vi "FB_MFA_SetMotorFeedback_Type1.vi"(11 "SetMotorFeedbackType":i16) -> (2 "MotorFeedback":i16, 3 "MotFbError":bool)   [LabVIEW 2011]
panel:
  out "error MotorFeedbackGet":errorcluster
  out "error MotorFeedBackPut":errorcluster
  out "AAABuild":i32
  in  "MintController":refnum<k7>(container)
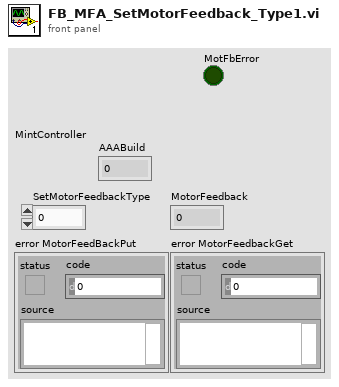
[diagram p1: front panel]
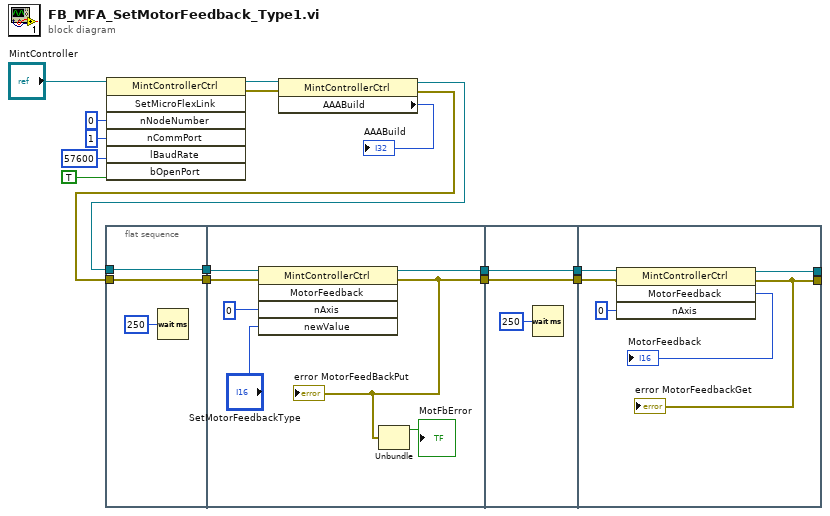
[diagram p0: block diagram]
diagram:
  n1 = flat-sequence {
    tunnel: [w19] -> w6
    tunnel: [w18] -> w5
    tunnel: w8 -> [w19]
    tunnel: w7 -> [w18]
    tunnel: w6 -> [w25]
    tunnel: w5 -> [w24]
    tunnel: [w23] -> w4
    tunnel: [w21] -> w3
    tunnel: w4 -> [w29]
    tunnel: w3 -> [w28]
    tunnel: [w29] -> w2
    tunnel: [w28] -> w1
    tunnel: w2 -> [w35]
    tunnel: w1 -> [w34]
    tunnel: [w31] -> _
    tunnel: [w30] -> _
    frame #0 {
      n2 = Wait (ms)(milliseconds to wait=u32 250) -> ()  [unwired: 1 out]
    }
    frame #1 {
      n3 = invoke class="MintControllerCtrl" method="MotorFeedback"(reference=w24, error in=w25, "nAxis"=i16 0, "newValue"="SetMotorFeedbackType") -> (reference out=w23:refnum<k7>, error out=w21:errorcluster)  [unwired: 1 in, 3 out]
      "error MotorFeedBackPut" <- w21
      n4 = Unbundle(w21) -> ("status"=→"MotFbError":bool)  [unwired: 2 out]
    }
    frame #2 {
      n5 = Wait (ms)(milliseconds to wait=u32 250) -> ()  [unwired: 1 out]
    }
    frame #3 {
      n6 = invoke class="MintControllerCtrl" method="MotorFeedback"(reference=w35, error in=w34, "nAxis"=i16 0 ("nBank")) -> (reference out=w31:refnum<k7>, error out=w30:errorcluster, "MotorFeedback"=→"MotorFeedback":i16)  [unwired: 1 in, 1 out]
      "error MotorFeedbackGet" <- w30
    }
  }
  n7 = invoke class="MintControllerCtrl" method="SetMicroFlexLink"(reference="MintController", "nNodeNumber"=i16 0, "nCommPort"=i16 1, "lBaudRate"=57600, "bOpenPort"=TRUE) -> (reference out=w16:refnum<k7>, error out=w10:errorcluster)  [unwired: 2 in, 5 out]
  n8 = property class="MintControllerCtrl"(reference=w16, error in=w10) -> (reference out=w7:refnum<k7>, error out=w8:errorcluster, "AAABuild"=→"AAABuild":i32)
